vi "DQMH System Message - Ready for Display.vi"(10 "Main VI Reference":refnum<vi>) -> (1 "Payload":variant, 2 "Identifier":string="Ready for Display", 5 "Source":T1)   [LabVIEW 2014, in "hse-dqmh.lvlib"]
uses:
  hse-dqmh.lvlib
  Controls/System Message Source.ctl
  Controls/System Message Framework Identifiers.ctl
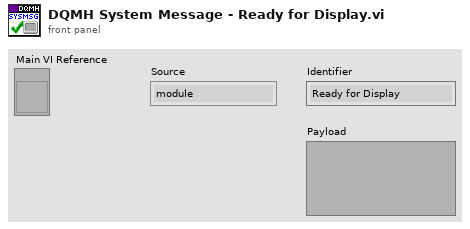
[diagram p1: front panel]
types:
  T1 = typedef "hse-dqmh.lvlib/System Message Source.ctl" = enum16{"module", "application", "network"}
  T2 = typedef "hse-dqmh.lvlib/System Message Framework Identifiers.ctl" = enum16{"Add to Run-Time Menu", "Ready for Display", "Removed from Subpanel"}
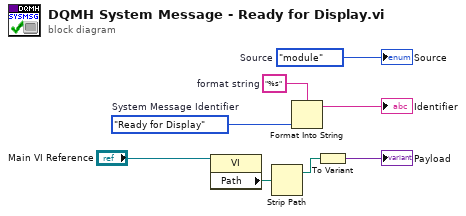
[diagram p0: block diagram]
diagram:
  w3 = "%s"  # format string
  w2 = System_Message_Framework_Identifiers."Ready for Display"  # System Message Identifier
  w8 = System_Message_Source."module"  # Source
  n1 = property class="VI"(reference="Main VI Reference") -> ("Path"=w5:path)  [unwired: 1 in, 2 out]
  n2 = Strip Path(path=w5) -> (stripped path=w4:path)  [unwired: 1 out]
  n3 = Format Into String(format string=w3, w2) -> (resulting string=→"Identifier":string)  [unwired: 2 in, 1 out]
  n4 = To Variant(anything=w4) -> (Variant=→"Payload":variant)
  "Source" <- w8
